vi "Numeric String to Array.vi"(8 "Sheet String":string) -> (2 "Table Array":dbl[](array[numeric]))   [LabVIEW 2018, in "Agilent U2000 Series.lvlib"]
doc: "Parses the sheet format string returned by instrument to an array of numeric."
uses:
  Agilent U2000 Series.lvlib
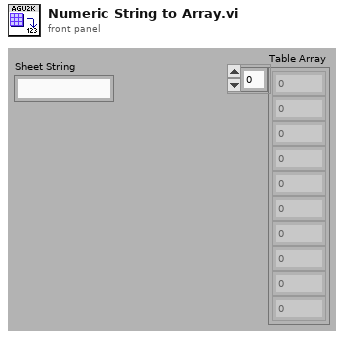
[diagram p1: front panel]
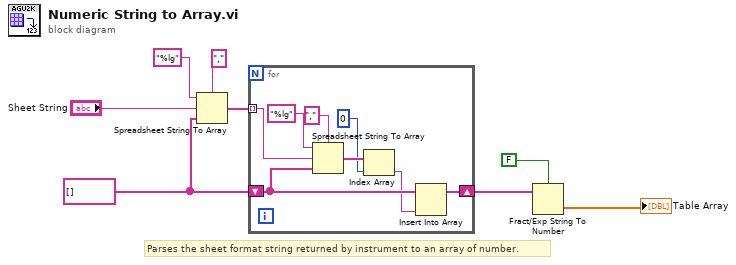
[diagram p0: block diagram]
diagram:
  w5 = string[] []
  # "Parses the sheet format string returned by instrument to an array of number."
  n1 = Spreadsheet String To Array(delimiter (Tab)=",", format string="%lg", spreadsheet string="Sheet String", array type (2D Dbl)=w5) -> (array=w6:string[])
  n2 = for {
    tunnel: w6 -> [w10] mode=indexing
    shift-right: [w16] -> w3
    shift-left: w5 -> [w14]
    n3 = Spreadsheet String To Array(delimiter (Tab)=",", format string="%lg", spreadsheet string=w10, array type (2D Dbl)=w14) -> (array=w13:string[])
    n4 = Index Array(array=w13, index=0) -> (element=w11:string)
    n5 = Insert Into Array(array=w14, new element=w11) -> (w16:string[])  [unwired: 1 in]
  }
  n6 = Fract/Exp String To Number(use system decimal point (T)=FALSE, string=w3) -> (number=→"Table Array":dbl[])  [unwired: 2 in, 1 out]
